vi "testVI.vi"() -> ()   [LabVIEW 2012]
uses:
  <vilib>/DAQmx/read.llb/DAQmx Read (Analog 2D DBL NChan NSamp).vi
  <vilib>/Analysis/Matrix/NI_Matrix.lvlib
  <vilib>/Analysis/Matrix/Numeric/Conversions/Matrix To Array - RM.vi
panel:
  in  "Resistansen":dbl
  in  "Spänningsintervall, slutpunkt":dbl
  in  "Spänningsintervall, startpunkt":dbl
  in  "Solcellens area":dbl(slide) scale=0.0..10.0
  in  "Antal mätpunkter":dbl
  in  "Välj typ av mätning":bool
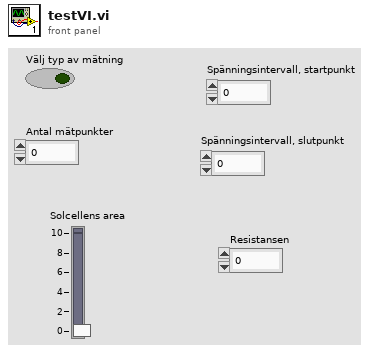
[diagram p1: front panel]
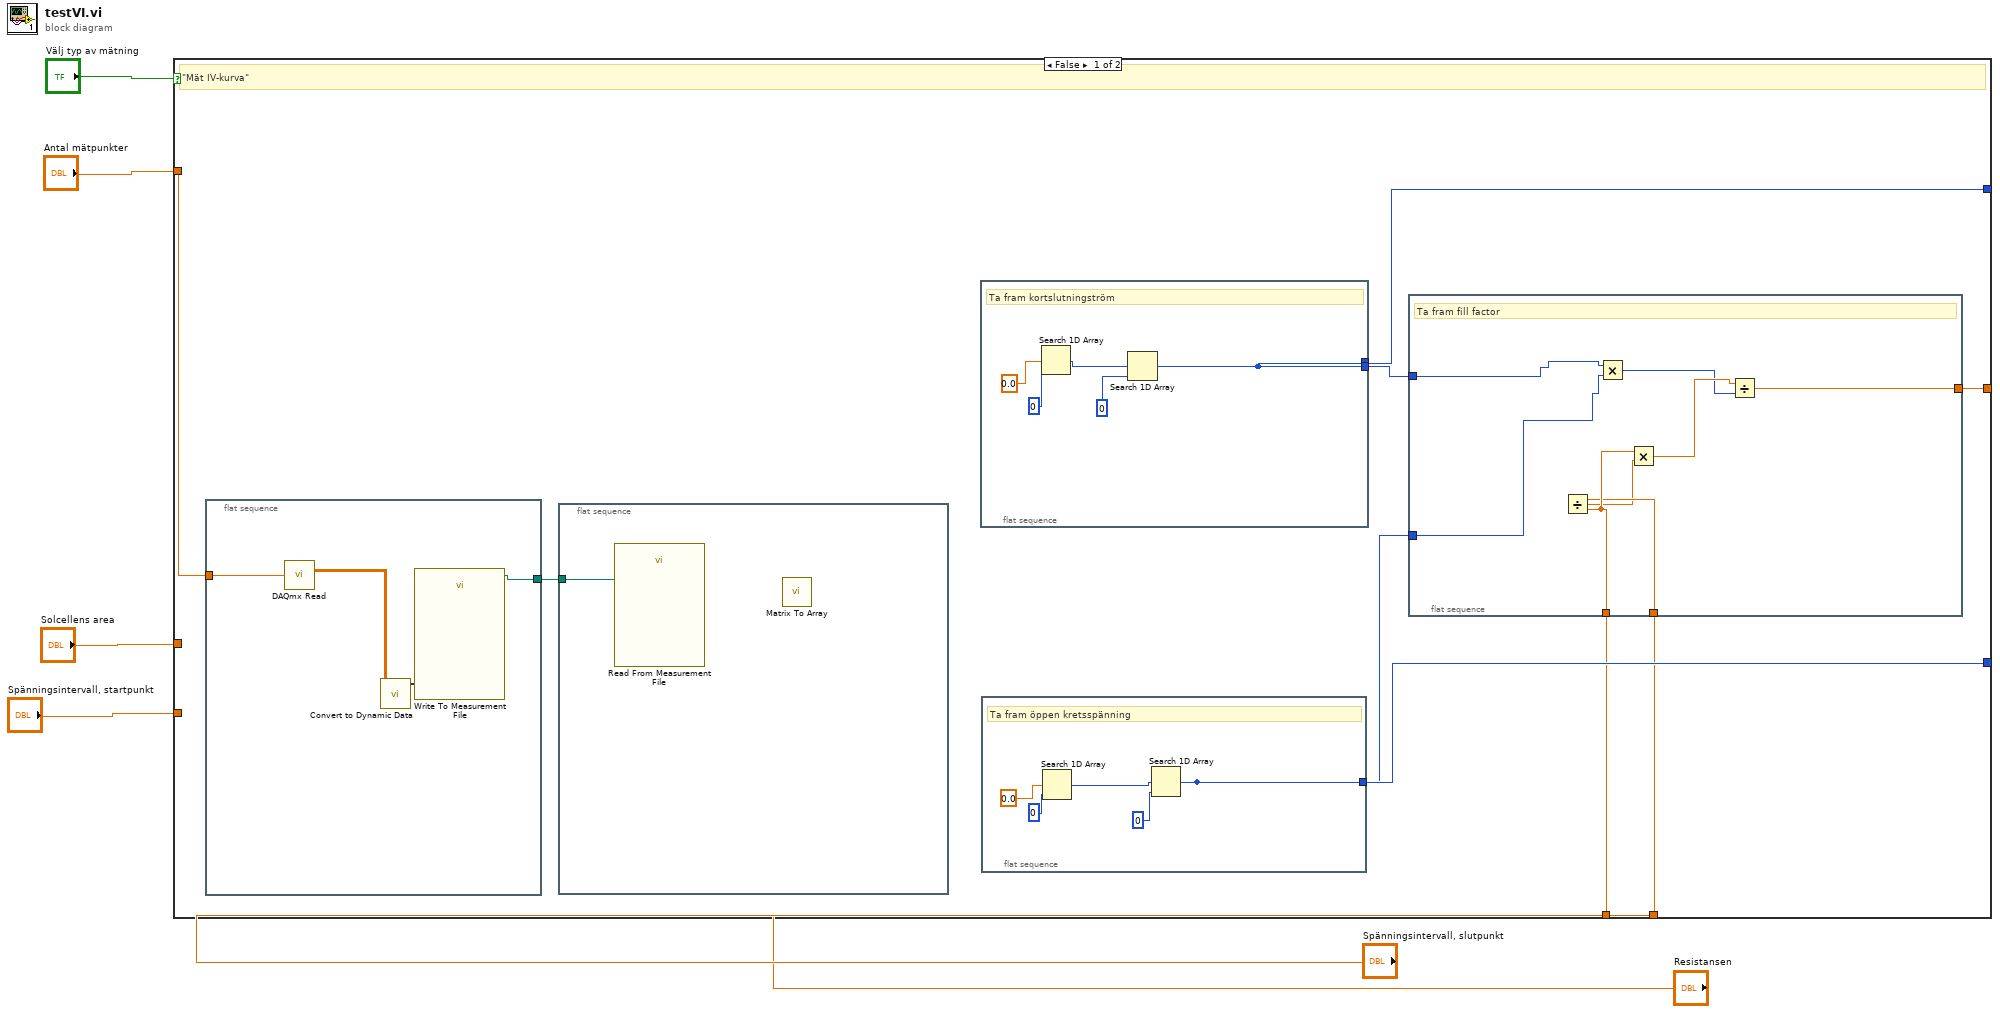
[diagram p0: block diagram]
diagram:
  n1 = case shown="False" "Välj typ av mätning" {
    tunnel: "Antal mätpunkter" -> [w15 _]
    tunnel: "Solcellens area" -> [_ _]
    tunnel: "Spänningsintervall, startpunkt" -> [_ _]
    tunnel: "Spänningsintervall, slutpunkt" -> [w9 _]
    tunnel: [w13 _] -> _
    tunnel: [w12 _] -> _
    tunnel: "Resistansen" -> [w8 _]
    tunnel: [w7 _] -> _
    frame False {
      # "\"Mät IV-kurva\""
      n2 = flat-sequence {
        tunnel: w15 -> [w37]
        tunnel: [w34] -> w14
        frame #0 {
          n3 = call-poly <vilib>:"DAQmx Read.vi"("number of samples per channel"=w37) -> ("data"=w36:dbl[][])  [unwired: 12 in, 2 out]
          n4 = call "Convert to Dynamic Data"("2D Array"=w36) -> ("Dynamic Data Type"=w35:dynamicdata)  [unwired: 3 in]
          n5 = call "Write To Measurement File"("Signals"=w35) -> ("Filename Out"=w34:path)  [unwired: 16 in, 2 out]
        }
      }
      n6 = flat-sequence {
        tunnel: w14 -> [w38]
        frame #0 {
          n7 = call "Read From Measurement File"("Filename"=w38) -> ()  [unwired: 5 in, 6 out]
          n8 = call-poly <vilib>:"Matrix To Array.vi"() -> ()  [unwired: 1 in, 1 out]
        }
      }
      n9 = flat-sequence {
        tunnel: [w29] -> w12
        tunnel: [w29] -> w11
        frame #0 {
          # "Ta fram kortslutningström"
          n10 = Search 1D Array(element=0.0, start index (0)=0) -> (index of element=w30:i32)  [unwired: 1 in]
          n11 = Search 1D Array(element=w30, start index (0)=0) -> (index of element=w29:i32)  [unwired: 1 in]
        }
      }
      n12 = flat-sequence {
        tunnel: [w24] -> w13
        tunnel: [w24] -> w10
        frame #0 {
          # "Ta fram öppen kretsspänning"
          n13 = Search 1D Array(element=0.0, start index (0)=0) -> (index of element=w28:i32)  [unwired: 1 in]
          n14 = Search 1D Array(element=w28, start index (0)=0) -> (index of element=w24:i32)  [unwired: 1 in]
        }
      }
      n15 = flat-sequence {
        tunnel: w11 -> [w18]
        tunnel: w10 -> [w17]
        tunnel: w9 -> [w23]
        tunnel: w8 -> [w22]
        tunnel: [w16] -> w7
        frame #0 {
          # "Ta fram fill factor"
          n16 = Divide(x=w22, y=w23) -> (x/y=w21:dbl)
          n17 = Multiply(x=w18, y=w17) -> (x*y=w19:i32)
          n18 = Multiply(x=w23, y=w21) -> (x*y=w20:dbl)
          n19 = Divide(x=w20, y=w19) -> (x/y=w16:dbl)
        }
      }
    }
    frame True {
    }
  }
